vi "Show Advanced Tab Write.vi"(4 "error in (no error)":errorcluster, 5 "Value":bool, 6 "Container State":T2, 7 "Display State In":T1={"Update"=FALSE, "Show advanced"=FALSE, "Fs (Hz)"=100000.0, "Show persist"=FALSE}) -> (0 "error out":errorcluster, 3 "Display State Out":T1={"Update"=FALSE, "Show advanced"=FALSE, "Fs (Hz)"=100000.0, "Show persist"=FALSE})   [LabVIEW 2020, in "Stimulus Channel (Full).xctl"]
uses:
  Stimulus Channel (Full).xctl
  <vilib>/_xctls/Container State.ctl
  State.ctl
  <vilib>/_xctls/XControlSupport.lvlib
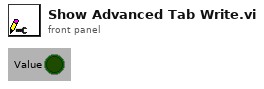
[diagram p1: front panel]
types:
  T1 = typedef "Stimulus Channel (Full).xctl/State.ctl" = cluster{"Update":bool, "Show advanced":bool, "Fs (Hz)":dbl, "Show persist":bool}
  T2 = typedef "XControlSupport.lvlib/Container State.ctl" = cluster{"Indicator?":bool, "Run Mode?":bool, " Refnum":refnum<vi>}
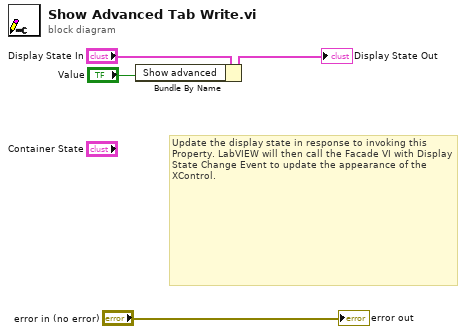
[diagram p0: block diagram]
diagram:
  # "Update the display state in response to invoking this Property. LabVIEW will then call the Facade VI with Display State Change Event to update the appearance of the XControl."
  n1 = Bundle By Name(cluster="Display State In", "Show advanced"="Value") -> (→"Display State Out":T1)
  "error out" <- "error in (no error)"
